vi "EnqueueEventLogger.vi"(6 "Priority":bool, 8 "Error In":errorcluster, 9 "Data":variant, 10 "Message":T1, 11 "EventLoggerQueue":refnum<queue>) -> (0 "Error Out":errorcluster, 3 "EventLoggerQueue out":refnum<queue>)   [LabVIEW 2019, in "EventLogger.lvlib"]
uses:
  Cluster - MessageCluster.ctl
  Enum - Message.ctl
  EventLogger.lvlib
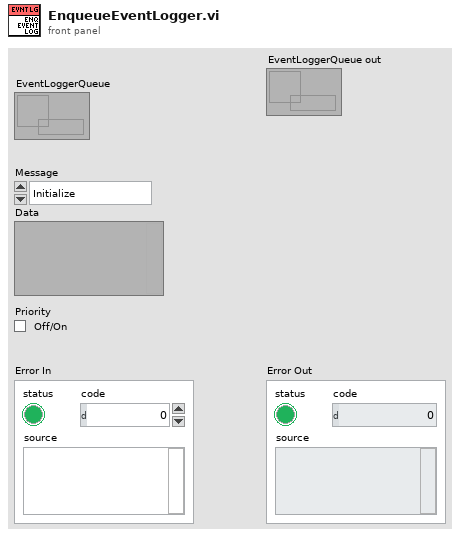
[diagram p1: front panel]
types:
  T1 = typedef "EventLogger.lvlib/Enum - Message.ctl" = enum16{"Initialize", "Idle", "CreateLog", "LogStrEvent", "LogErrorEvent", "LogVICall", "Error", "Exit"}
  T2 = typedef "EventLogger.lvlib/Cluster - MessageCluster.ctl" = cluster{"Message":T1, "Data":variant}
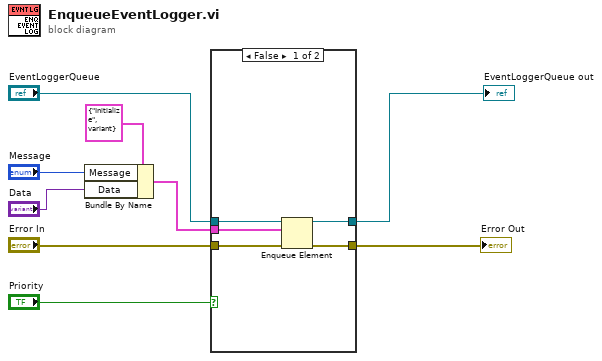
[diagram p0: block diagram]
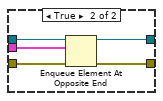
[diagram p2: hidden frame]
diagram:
  n1 = Bundle By Name(cluster=T2 {"Message"=enum."Initialize", "Data"=variant} ("element"), "Message"="Message", "Data"="Data") -> (w4:T2)
  n2 = case shown="False" "Priority" {
    tunnel: "Error In" -> [w14 w19]
    tunnel: [w13 w18] -> w8
    tunnel: "EventLoggerQueue" -> [w12 w17]
    tunnel: [w11 w16] -> w6
    tunnel: w4 -> [w10 w15]
    frame False {
      n3 = Enqueue Element(queue=w12, element=w10, error in (no error)=w14) -> (queue out=w11:refnum<queue>, error out=w13:errorcluster)  [unwired: 1 in, 1 out]
    }
    frame True {
      n4 = Enqueue Element At Opposite End(queue=w17, element=w15, error in (no error)=w19) -> (queue out=w16:refnum<queue>, error out=w18:errorcluster)  [unwired: 1 in, 1 out]
    }
  }
  "Error Out" <- w8
  "EventLoggerQueue out" <- w6
